vi "RPC Open VI Reference.vi"(8 "error in (no error)":errorcluster, 10 "VI path (empty)":path, 11 "app reference (empty)":refnum<vi>) -> (0 "error out":errorcluster, 2 "vi reference":refnum<vi>, 3 "dup app reference":refnum<vi>)   [LabVIEW 2011]
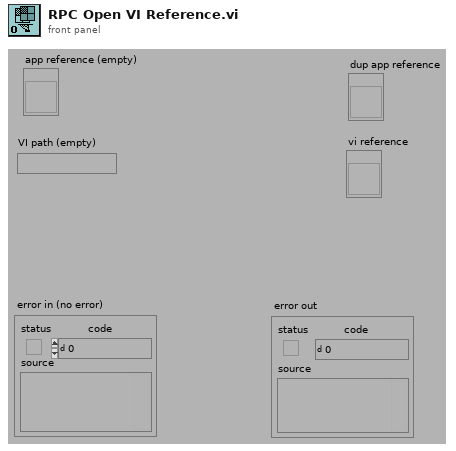
[diagram p1: front panel]
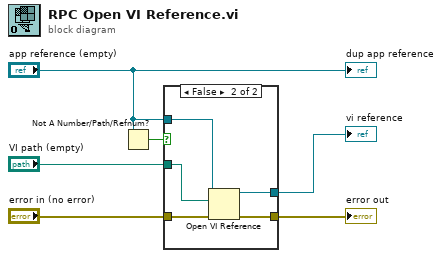
[diagram p0: block diagram]
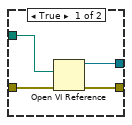
[diagram p2: hidden frame]
diagram:
  n1 = Not A Number/Path/Refnum?(number/path/refnum="app reference (empty)") -> (NaN/Path/Refnum?=w6:bool)
  n2 = case shown="False" w6 {
    tunnel: "app reference (empty)" -> [_ w12]
    tunnel: "error in (no error)" -> [w10 w15]
    tunnel: [w9 w14] -> w3
    tunnel: [w8 w13] -> w1
    tunnel: "VI path (empty)" -> [w7 w11]
    frame True {
      n3 = Open VI Reference(vi path=w7, error in (no error)=w10) -> (vi reference=w8:refnum<vi>, error out=w9:errorcluster)  [unwired: 4 out]
    }
    frame False {
      n4 = Open VI Reference(application reference (local)=w12, vi path=w11, error in (no error)=w15) -> (vi reference=w13:refnum<vi>, error out=w14:errorcluster)  [unwired: 3 out]
    }
  }
  "error out" <- w3
  "vi reference" <- w1
  "dup app reference" <- "app reference (empty)"
